vi "CS_Contents_Main.vi"   [LabVIEW 2014]
doc: "This \"contents\" VI contains all components of CS, which belong to the category \"Main\". Everything in here is vital for running CS."
uses:
  CSClass/CSCore/GUIs/GeneralObjectGUI/GeneralObjectGUI.lvlib
  CSClass/CSCore/ObjectInspector/ObjectInspector.lvlib
  CSClass/CSCore/CSAccessSystem/CSAccessClient/CSAccessClient.lvlib
  CSClass/CSCore/CSAccessSystem/CSAccessViewer/CSAccessViewer.lvlib
  CSClass/CSCore/CSSystem/CSSystemLib/CSSystemLib.lvlib
  CSClass/CSCore/CSObj/CSObj.lvlib
  CSClass/CSCore/BaseSM/BaseSM.lvlib
  CSClass/CSCore/CAEObj/CAEObj.lvlib
  CSClass/CSCore/BaseProcess/BaseProcess.lvlib
  CSClass/CSCore/NotifierObj/NotifierObj.lvlib
  CSClass/CSCore/SuperProc/SuperProc.lvlib
  CSClass/CSCore/BaseGUI/BaseGUI.lvlib
  CSClass/CSCore/GUIs/DIMGUIs/DIMHistogramGUI/DIMHistogramGUI.lvlib
  CSClass/CSCore/GUIs/DIMGUIs/DIMTrendGUI/DIMTrendGUI.lvlib
  CSClass/CSCore/GUIs/DIMGUIs/DIMTableView/DIMTableView.lvlib
  CSClass/CSCore/CSTimer/CSTimer.lvlib
  CSClass/CSCore/GUIs/CSPopUpMsgBox/CSPopUpMsgBox.lvlib
  CSClass/CSCore/CSSimulation/SimMCS/SimMCS.lvlib
  CSClass/CSCore/CSSimulation/SimMotor/SimMotor.lvlib
  CSClass/CSCore/CSSimulation/SimDigiIO/SimDigiIO.lvlib
  CSClass/CSCore/CSSimulation/SimAFG/SimAFG.lvlib
  CSClass/CSCore/CSSimulation/SimPowerSupply/SimPowerSupply.lvlib
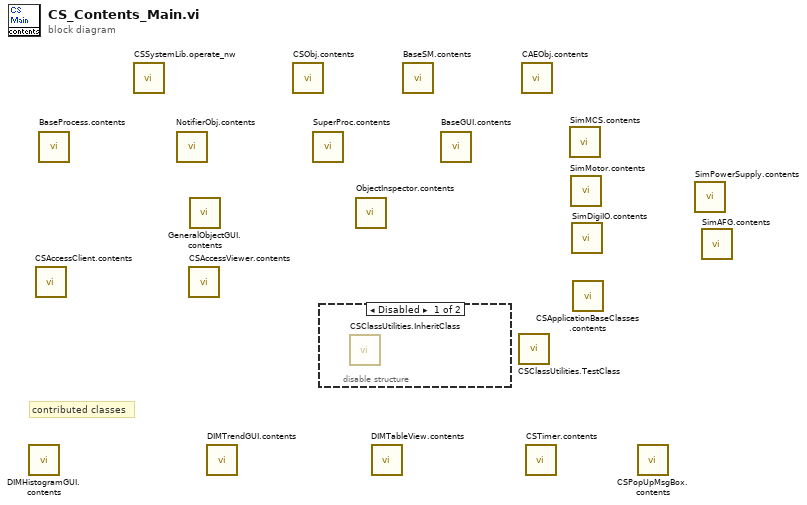
[diagram p0: block diagram]
diagram:
  # "contributed classes"
  n1 = call "DIMHistogramGUI.contents.vi"() -> ()  [unwired: 1 in]
  n2 = call "CSAccessClient.contents.vi"() -> ()  [unwired: 1 in]
  n3 = call "BaseProcess.contents.vi"() -> ()  [unwired: 1 in]
  n4 = call "CSSystemLib.operate_nw.vi"() -> ()  [unwired: 20 in]
  n5 = call "NotifierObj.contents.vi"() -> ()  [unwired: 1 in]
  n6 = call "CSAccessViewer.contents.vi"() -> ()  [unwired: 1 in]
  n7 = call "GeneralObjectGUI.contents.vi"() -> ()  [unwired: 1 in]
  n8 = call "DIMTrendGUI.contents.vi"() -> ()  [unwired: 1 in]
  n9 = call "CSObj.contents.vi"() -> ()  [unwired: 1 in]
  n10 = call "SuperProc.contents.vi"() -> ()  [unwired: 1 in]
  n11 = disable-structure shown="Disabled" {
    frame Disabled {
      n12 = call "CSClassUtilities.InheritClass.vi"() -> ()  [unwired: 1 in]
    }
    frame Enabled {
    }
  }
  n13 = call "ObjectInspector.contents.vi"() -> ()  [unwired: 1 in]
  n14 = call "DIMTableView.contents.vi"() -> ()  [unwired: 1 in]
  n15 = call "BaseSM.contents.vi"() -> ()  [unwired: 1 in]
  n16 = call "BaseGUI.contents.vi"() -> ()  [unwired: 1 in]
  n17 = call "CSClassUtilities.TestClass.vi"() -> ()  [unwired: 20 in]
  n18 = call "CAEObj.contents.vi"() -> ()  [unwired: 1 in]
  n19 = call "CSTimer.contents.vi"() -> ()  [unwired: 1 in]
  n20 = call "SimMCS.contents.vi"() -> ()  [unwired: 1 in]
  n21 = call "SimMotor.contents.vi"() -> ()  [unwired: 1 in]
  n22 = call "SimDigiIO.contents.vi"() -> ()  [unwired: 1 in]
  n23 = call "CSApplicationBaseClasses.contents.vi"() -> ()  [unwired: 1 in]
  n24 = call "CSPopUpMsgBox.contents.vi"() -> ()  [unwired: 1 out]
  n25 = call "SimPowerSupply.contents.vi"() -> ()  [unwired: 1 in]
  n26 = call "SimAFG.contents.vi"() -> ()  [unwired: 1 in]
